vi "Get Session Info - 1Pin 1Sess .vi"(8 "error in":errorcluster, 10 "pin or relay name":string, 11 "session reservation in":refnum<class "Session Reservation.lvclass">) -> (0 "error out":errorcluster, 2 "session info":T1, 3 "session reservation out":refnum<class "Session Reservation.lvclass">)   [LabVIEW 2020, in "MeasurementLink Session Management.lvlib" / "Session Reservation.lvclass"]
doc: "Gets the connection information for the given <b>pin type</b>, <b>pin or relay name</b>, <b>instrument</b>, and <b>site</b>.The <b>instrument</b> input must return a valid instrument_type_id from the <b>Get Instrument Type ID.vi</b> override. The <b>connection type</b> input should be a cluster with two elements. The first element is a <b>Connection.ctl</b> cluster. The second element is the type of the session."
uses:
  Session Reservation.lvclass
  MeasurementLink Session Management Client/RPC Messages/ni_measurementlink_sessionmanagement_v1_SessionInformation.ctl
  MeasurementLink Session Management Client/RPC Messages/nidevice_grpc_Session.ctl
  MeasurementLink Session Management Client/RPC Messages/ni_measurementlink_sessionmanagement_v1_ChannelMapping.ctl
  Session Reservation.lvclass/Session Reservation.ctl
  Is DVR Valid.vi
  MeasurementLink Measurement Server/Helpers/Error Strings Global Internal.vi
  MeasurementLink Session Management Client/MeasurementLink Session Management Client.lvlib
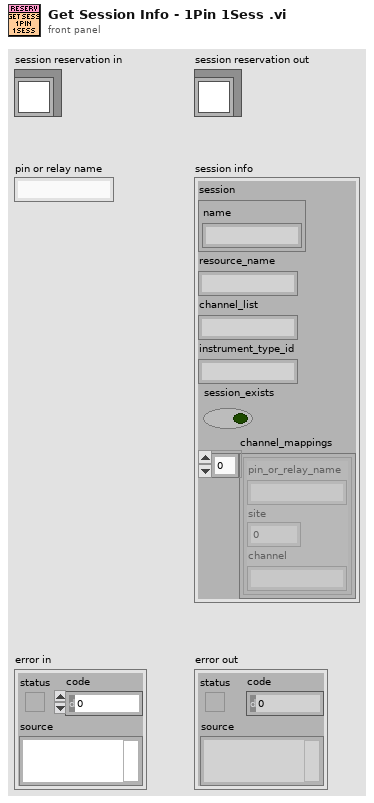
[diagram p1: front panel]
types:
  T1 = typedef "MeasurementLink Session Management Client.lvlib/ni_measurementlink_sessionmanagement_v1_SessionInformation.ctl" = cluster{"session":T2, "resource_name":string, "channel_list":string, "instrument_type_id":string, "session_exists":bool, "channel_mappings":T3[]}
  T2 = typedef "MeasurementLink Session Management Client.lvlib/nidevice_grpc_Session.ctl" = cluster{"name":string}
  T3 = typedef "MeasurementLink Session Management Client.lvlib/ni_measurementlink_sessionmanagement_v1_ChannelMapping.ctl" = cluster{"pin_or_relay_name":string, "site":i32, "channel":string}
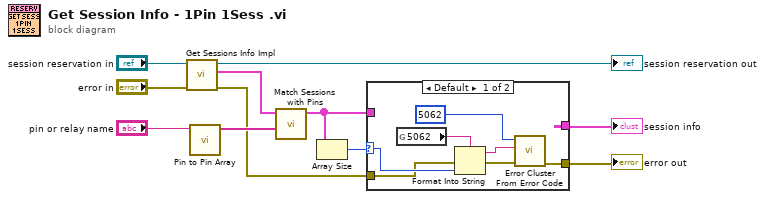
[diagram p0: block diagram]
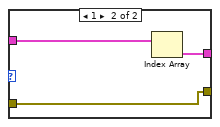
[diagram p2: hidden frame]
diagram:
  n1 = call "Get Sessions Info Impl.vi"("error in"="error in", "session reservation in"="session reservation in") -> ("error out"=w3:errorcluster, "sessions info"=w7:T1[], "session reservation out"=→"session reservation out":refnum<class "Session Reservation.lvclass">)  [unwired: 7 in]
  n2 = call "Pin to Pin Array.vi"("pin or relay name"="pin or relay name") -> ("pin array"=w6:string[])  [unwired: 10 in]
  n3 = call "Match Sessions with Pins.vi"("pin array"=w6, "Sessions Info In"=w7) -> ("Sessions Info Out"=w4:T1[])  [unwired: 9 in]
  n4 = Array Size(array=w4) -> (size(s)=w1:i32)
  n5 = case shown="Default" w1 {
    selector: w1 -> [w13 _]
    tunnel: w4 -> [_ w21]
    tunnel: [_ w20] -> w5
    tunnel: [w18 w19] -> w2
    tunnel: w3 -> [w12 w19]
    frame Default {
      n6 = global read "Error Strings Global Internal.vi" "5062"() -> (w14:string)
      n7 = Format Into String(format string=w14, error in=w12, w13) -> (resulting string=w15:string, error out=w16:errorcluster)  [unwired: 1 in]
      n8 = call <vilib>:"Error Cluster From Error Code.vi"("error in (no error)"=w16, "error message (\"\")"=w15, "error code (0)"=5062) -> ("error out"=w18:errorcluster)  [unwired: 6 in]
    }
    frame 1 {
      n9 = Index Array(array=w21) -> (element=w20:T1)  [unwired: 1 in]
    }
  }
  "error out" <- w2
  "session info" <- w5
